vi "Test Invalid Write - Server Error.vi"() -> ()   [LabVIEW 2024]
uses:
  Mock Sift Proxy Server/Mock Sift Proxy Server.lvclass
  Sift API/Sift Client.lvclass
  Sift API/Types/Data Type.ctl
  Sift Client.lvlib
panel:
  out "Server Error":errorcluster
  out "Success 2":bool
  out "Error 2":errorcluster
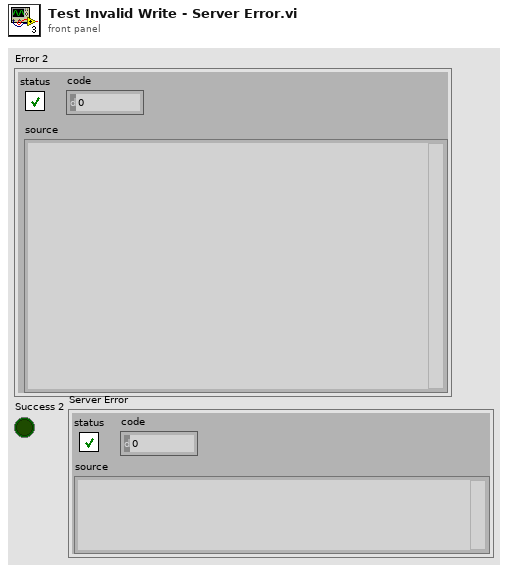
[diagram p1: front panel]
types:
  T1 = typedef "Sift Client.lvlib/Data Type.ctl" = enum8{"double", "float", "uint64", "int64", "uint32", "int32", "bool", "bit field", "enum"}
  T2 = typedef "Sift Client.lvlib/Timestamp.ctl" = cluster{"seconds":i64, "nanos":i32}
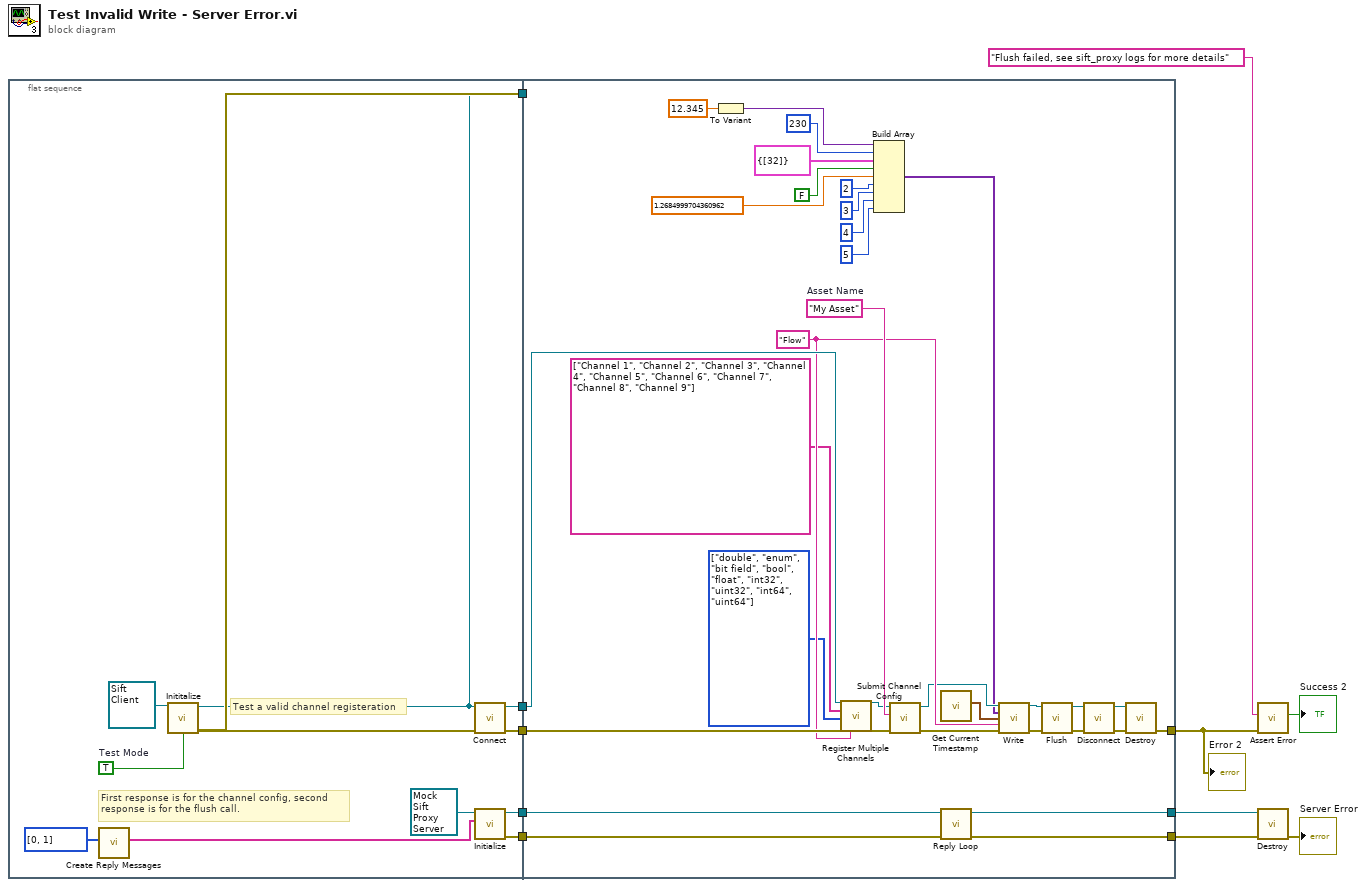
[diagram p0: block diagram]
diagram:
  n1 = flat-sequence {
    tunnel: [w22] -> w12
    tunnel: [w19] -> w11
    tunnel: [w18] -> w10
    tunnel: [w17] -> w9
    tunnel: [w16] -> w8
    tunnel: [w15] -> w7
    tunnel: [w51] -> w6
    tunnel: w12 -> [w52]
    tunnel: [w55] -> w2
    tunnel: w11 -> [_]
    tunnel: w10 -> [_]
    tunnel: w9 -> [w50]
    tunnel: w8 -> [w49]
    tunnel: w7 -> [w46]
    tunnel: [w45] -> w5
    frame #0 {
      w20 = TRUE  # Test Mode
      # "First response is for the channel config, second\nresponse is for the flush call."
      # "Test a valid channel registeration"
      n2 = call "Create Reply Messages.vi"("Replies"=u8[] [0, 1]) -> ("String Replies"=w13:string[])  [unwired: 10 in]
      n3 = call-dynamic "Inititalize.vi"("Sift Client in"=refnum<class "Sift Client.lvclass"> refnum ("Sift Client.lvlib:Sift Client.lvclass"), "Test Mode"=w20) -> ("Sift Client out"=w18:refnum<class "Sift Client.lvclass">, "error out"=w19:errorcluster)  [unwired: 12 in]
      n4 = call-dynamic "Connect.vi"("error in (no error)"=w19, "Sift Client in"=w18) -> ("error out"=w17:errorcluster, "Sift Client out"=w16:refnum<class "Sift Client.lvclass">)  [unwired: 7 in, 1 out]
      n5 = call-dynamic "Initialize.vi"("Mock Replies"=w13, "Mock Sift Proxy Server in"=refnum<class "Mock Sift Proxy Server.lvclass"> refnum ("Mock Sift Proxy Server.lvclass")) -> ("error out"=w15:errorcluster, "Mock Sift Proxy Server out"=w22:refnum<class "Mock Sift Proxy Server.lvclass">)  [unwired: 8 in]
    }
    frame #1 {
      w39 = T1[] [enum."double", enum."enum", enum."bit field", enum."bool", enum."float", enum."int32", enum."uint32", enum."int64", enum."uint64"] items=["double", "float", "uint64", "int64", "uint32", "int32", "bool", "bit field", "enum"]
      w54 = "My Asset"  # Asset Name
      w43 = "Flow" ("Flow Name")
      n6 = To Variant(anything=12.345) -> (Variant=w38:variant)
      n7 = call "Register Multiple Channels.vi"("Sift Client in"=w49, "Names"=string[] ["Channel 1", "Channel 2", "Channel 3", "Channel 4", "Channel 5", "Channel 6", "Channel 7", "Channel 8", "Channel 9"], "Data Types"=w39, "error in (no error)"=w50, "Flow Name"=w43) -> ("Sift Client out"=w53:refnum<class "Sift Client.lvclass">, "error out"=w56:errorcluster)  [unwired: 21 in]
      n8 = Build Array(w38, 230, cluster{u8[]} {[32]}, FALSE, sgl 1.2685, 2, 3, 4, 5) -> (w28:variant[])
      n9 = call-dynamic "Submit Channel Config.vi"("error in (no error)"=w56, "Asset Name"=w54, "Sift Client in"=w53) -> ("error out"=w41:errorcluster, "Sift Client out"=w42:refnum<class "Sift Client.lvclass">)  [unwired: 7 in]
      n10 = call "Get Current Timestamp.vi"() -> ("Timestamp"=w44:T2)  [unwired: 11 in]
      n11 = call-dynamic "Reply Loop.vi"("error in (no error)"=w46, "Mock Sift Proxy Server in"=w52) -> ("error out"=w45:errorcluster, "Mock Sift Proxy Server out"=w51:refnum<class "Mock Sift Proxy Server.lvclass">)  [unwired: 8 in]
      n12 = call-dynamic "Write.vi"("Sift Client in"=w42, "Values"=w28, "Timestamp"=w44, "Flow Name"=w43, "error in (no error)"=w41) -> ("Sift Client out"=w27:refnum<class "Sift Client.lvclass">, "error out"=w25:errorcluster)  [unwired: 9 in]
      n13 = call-dynamic "Flush.vi"("error in (no error)"=w25, "Sift Client in"=w27) -> ("error out"=w24:errorcluster, "Sift Client out"=w26:refnum<class "Sift Client.lvclass">)  [unwired: 7 in, 1 out]
      n14 = call-dynamic "Disconnect.vi"("error in (no error)"=w24, "Sift Client in"=w26) -> ("error out"=w47:errorcluster, "Sift Client out"=w48:refnum<class "Sift Client.lvclass">)  [unwired: 8 in]
      n15 = call-dynamic "Destroy.vi"("error in (no error)"=w47, "Sift Client in"=w48) -> ("error out"=w55:errorcluster)  [unwired: 8 in, 1 out]
    }
  }
  n16 = call "Assert Error.vi"("Error"=w2, "Error String"="Flush failed, see sift_proxy logs for more details") -> ("Success"=→"Success 2":bool)  [unwired: 9 in]
  n17 = call-dynamic "Destroy.vi"("error in (no error)"=w5, "Mock Sift Proxy Server in"=w6) -> ("error out"=→"Server Error":errorcluster)  [unwired: 8 in, 1 out]
  "Error 2" <- w2
